vi "RSZVB Set Frequency Conversion Type.vi"(8 "error in (no error)":errorcluster {"code" format="%.0x"}, 10 "Converter Type (ZVA-Z110)":string="ZVA-Z110", 11 "VISA session":refnum<visa-resource-name>) -> (0 "error out":errorcluster {"code" format="%.0x"}, 3 "dup VISA session":refnum<visa-resource-name>)   [LabVIEW 2011]
doc: "This VI selects the frequency converter type for enhanced frequency-converting measurements (with option ZVA-K8, Enhanced Frequency Conversion). \n\nNote(s):\n\n(1) This VI is available only on R&S ZVA and ZVT instrument.\n\nRemote-control command(s):\nSENSe<Ch>:FREQuency:CONVersion:DEVice:NAME '<Converter Type>'"
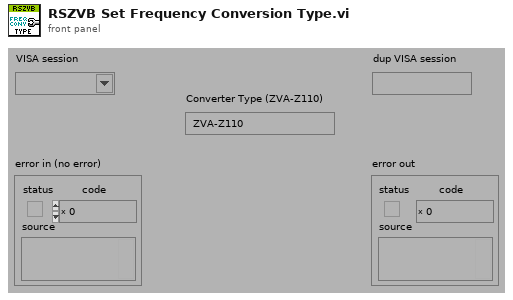
[diagram p1: front panel]
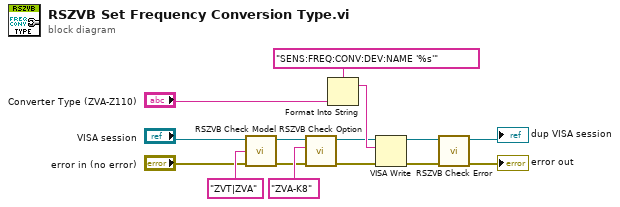
[diagram p0: block diagram]
diagram:
  n1 = call "RSZVB Check Model.vi"("error in (no error)"="error in (no error)", "Model"="ZVT|ZVA" ("Options"), "VISA session"="VISA session") -> ("error out"=w8:errorcluster, "dup VISA session"=w9:refnum<visa-resource-name>)  [unwired: 7 in]
  n2 = call "RSZVB Check Option.vi"("error in (no error)"=w8, "Options"="ZVA-K8", "VISA session"=w9) -> ("error out"=w6:errorcluster, "dup VISA session"=w7:refnum<visa-resource-name>)  [unwired: 7 in]
  n3 = Format Into String(format string="SENS:FREQ:CONV:DEV:NAME '%s'", "Converter Type (ZVA-Z110)") -> (resulting string=w12:string)  [unwired: 2 in, 1 out]
  n4 = VISA Write(VISA resource name=w7, write buffer=w12, error in (no error)=w6) -> (VISA resource name out=w13:refnum<visa-resource-name>, error out=w14:errorcluster)  [unwired: 1 out]
  n5 = call "RSZVB Check Error.vi"("error in (no error)"=w14, "VISA session"=w13) -> ("error out"=→"error out":errorcluster, "dup VISA session"=→"dup VISA session":refnum<visa-resource-name>)  [unwired: 8 in]
